vi "XW_Map_PreProc_wrapper_PN.vi"(4 "Domain padding factor":dbl=1.01, 6 "cap indicial sum to n":bool, 7 "XW_Calib_Map file path":path, 8 "surface order (n)":i32=3, 9 "Apply calibration corrections":bool=TRUE, 10 "Calib const":dbl[](array[numeric]) format="%.4f", 11 "Map method":T1=enum."Psi_eff, k = f(Umagn.)") -> ()   [LabVIEW 2010]
uses:
  XW calib map/Map method.ctl
  XW calib map/Qtree vis/Trimmed down TreeNode2D.ctl
  XW calib map/XW_Map_Global.vi
panel:
  out "All nodes processed and processed without error":bool
  # "For polysurface method only:"
  # "For trimesh method only:"
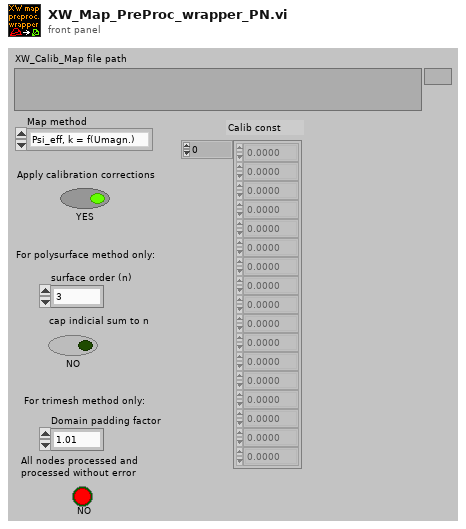
[diagram p1: front panel]
types:
  T1 = typedef "Map method.ctl" = enum16{"Triangle mesh", "Polynomial surface", "Const. Psi_eff (std.)", "Psi_eff = f(Umagn.)", "Psi_eff, k = f(Umagn.)"}
  T2 = cluster{"Calib const[0]":dbl, "Calib const[1]":dbl, "Calib const[2]":dbl, "Calib const[3]":dbl, "Calib const[4]":dbl, "Calib const[5]":dbl, "Calib const[6]":dbl, "Calib const[7]":dbl, "Calib const[8]":dbl, "Calib const[9]":dbl, "Calib const[10]":dbl, "Calib const[11]":dbl, "Calib const[12]":dbl, "Calib const[13]":dbl, "Calib const[14]":dbl, "Calib const[15]":dbl, "Calib const[16]":dbl, "Calib const[17]":dbl}
  T3 = typedef "Trimmed down TreeNode2D.ctl" = cluster{"Xmax":dbl, "Xmin":dbl, "Ymax":dbl, "Ymin":dbl, "Xc":dbl, "Yc":dbl, "ObjIndexList":i32[], "NodeQ1Index":i32, "NodeQ2Index":i32, "NodeQ3Index":i32, "NodeQ4Index":i32}
  T4 = typedef "Triangle2D.ctl" = cluster{"V10":dbl[], "V20":dbl[], "1/det":dbl, "V0":cluster{"PosVector":dbl[], "ValueVector":dbl[]}, "V1":cluster{"PosVector":dbl[], "ValueVector":dbl[]}, "V2":cluster{"PosVector":dbl[], "ValueVector":dbl[]}, "V21":dbl[]}
  T5 = typedef "TreeNode2D.ctl" = cluster{"Xmax":dbl, "Xmin":dbl, "Ymax":dbl, "Ymin":dbl, "Xc":dbl, "Yc":dbl, "Px":dbl, "Py":dbl, "q":dbl, "Level":i32, "ObjIndexList":i32[], "ParentIndex":i32, "NodeQ1Index":i32, "NodeQ2Index":i32, "NodeQ3Index":i32, "NodeQ4Index":i32, "EdgeVectorsQ1":dbl[][], "EdgeVectorsQ2":dbl[][], "EdgeVectorsQ3":dbl[][], "EdgeVectorsQ4":dbl[][], "PointOnEdgeVectorsQ1":dbl[][], "PointOnEdgeVectorsQ2":dbl[][], "PointOnEdgeVectorsQ3":dbl[][], "PointOnEdgeVectorsQ4":dbl[][]}
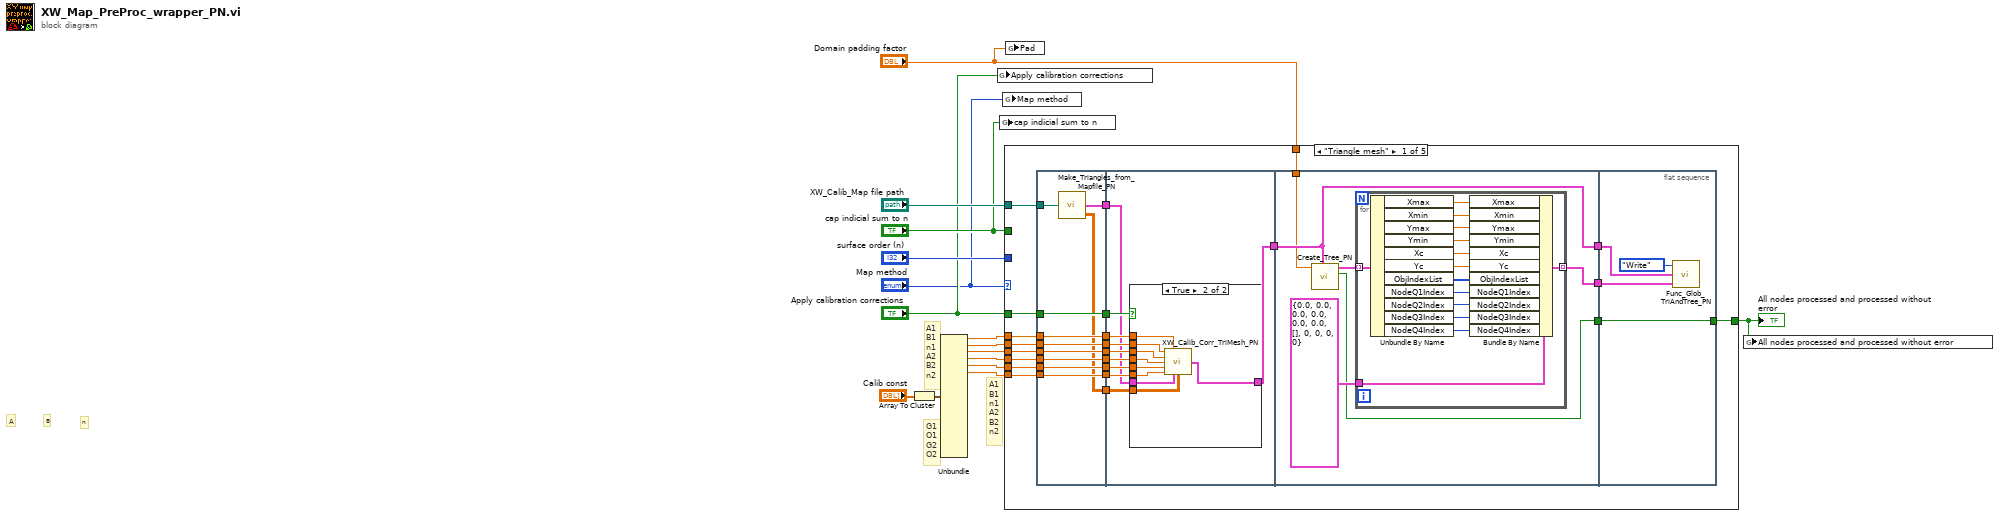
[diagram p0: block diagram]
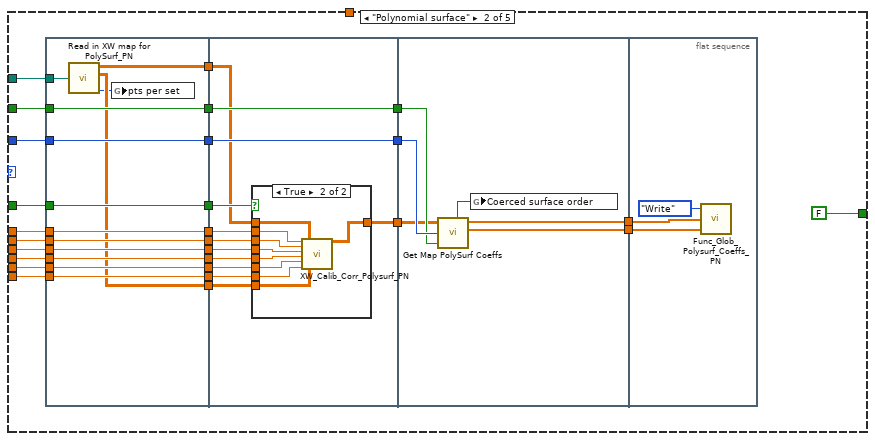
[diagram p3: hidden frame]
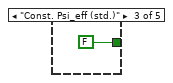
[diagram p5: hidden frame]
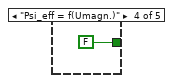
[diagram p6: hidden frame]
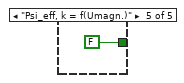
[diagram p7: hidden frame]
diagram:
  # "A1\nB1\nn1\nA2\nB2\nn2"
  # "G1\nO1\nG2\nO2"
  # "A1\nB1\nn1\nA2\nB2\nn2"
  # "n"
  # "B"
  # "A"
  n1 = Array To Cluster(array="Calib const") -> (cluster=w15:T2)
  n2 = Unbundle(w15) -> ("Calib const[0]"=w13:dbl, "Calib const[1]"=w12:dbl, "Calib const[2]"=w11:dbl, "Calib const[3]"=w10:dbl, "Calib const[4]"=w9:dbl, "Calib const[5]"=w8:dbl)  [unwired: 12 out]
  n3 = global write "XW_Map_Global.vi" "Apply calibration corrections"("Apply calibration corrections") -> ()
  n4 = global write "XW_Map_Global.vi" "cap indicial sum to n"("cap indicial sum to n") -> ()
  n5 = global write "XW_Map_Global.vi" "Map method"("Map method") -> ()
  n6 = case shown="\"Triangle mesh\"" "Map method" {
    tunnel: "Apply calibration corrections" -> [w38 w119 _ _ _]
    tunnel: w13 -> [w37 w118 _ _ _]
    tunnel: w12 -> [w36 w117 _ _ _]
    tunnel: w11 -> [w35 w116 _ _ _]
    tunnel: w10 -> [w34 w115 _ _ _]
    tunnel: w9 -> [w33 w114 _ _ _]
    tunnel: w8 -> [w32 w113 _ _ _]
    tunnel: "surface order (n)" -> [_ w112 _ _ _]
    tunnel: "cap indicial sum to n" -> [_ w111 _ _ _]
    tunnel: "XW_Calib_Map file path" -> [w31 w99 _ _ _]
    tunnel: [w23 FALSE FALSE ("All nodes processed and processed without error") FALSE ("All nodes processed and processed without error") FALSE ("All nodes processed and processed without error")] -> w1
    tunnel: "Domain padding factor" -> [w22 _ _ _ _]
    frame "Triangle mesh" {
      n7 = flat-sequence {
        tunnel: w31 -> [w41]
        tunnel: w32 -> [w42]
        tunnel: w33 -> [w43]
        tunnel: w34 -> [w44]
        tunnel: w35 -> [w45]
        tunnel: w36 -> [w46]
        tunnel: w37 -> [w47]
        tunnel: w38 -> [w48]
        tunnel: [w48] -> w30
        tunnel: [w47] -> w29
        tunnel: [w46] -> w28
        tunnel: [w45] -> w27
        tunnel: [w44] -> w26
        tunnel: [w43] -> w25
        tunnel: [w42] -> w24
        tunnel: [w40] -> w20
        tunnel: [w39] -> w16
        tunnel: w30 -> [w58]
        tunnel: w29 -> [w57]
        tunnel: w28 -> [w56]
        tunnel: w27 -> [w55]
        tunnel: w26 -> [w54]
        tunnel: w25 -> [w53]
        tunnel: w24 -> [w52]
        tunnel: w20 -> [w51]
        tunnel: [w50] -> w19
        tunnel: w16 -> [w49]
        tunnel: w22 -> [w69]
        tunnel: [w72] -> w21
        tunnel: w19 -> [w71]
        tunnel: [w71] -> w18
        tunnel: [w70] -> w17
        tunnel: [w92] -> w23
        tunnel: w21 -> [w92]
        tunnel: w18 -> [w91]
        tunnel: w17 -> [w90]
        frame #0 {
          n8 = call "Make_Triangles_from_Mapfile_PN.vi"("XW_Calib_Map file path (dialog if empty)"=w41) -> ("Triangles"=w40:T4[], "Zero angle dataset from map (used for calib. correction)"=w39:dbl[][])  [unwired: 1 out]
        }
        frame #1 {
          n9 = case shown="True" w58 {
            tunnel: w52 -> [_ w63]
            tunnel: w53 -> [_ w64]
            tunnel: w54 -> [_ w65]
            tunnel: w55 -> [_ w68]
            tunnel: w56 -> [_ w67]
            tunnel: w57 -> [_ w66]
            tunnel: w51 -> [w59 w62]
            tunnel: [w59 w61] -> w50
            tunnel: w49 -> [_ w60]
            frame False {
              # "if not correcting, then set\ncorrected tris equal to\noriginal tris for use"
            }
            frame True {
              n10 = call "XW_Calib_Corr_TriMesh_PN.vi"("B1 from Vel. Calib"=w67, "A1 from Vel. Calib"=w66, "n1 from Vel. Calib"=w68, "A2 from Vel. Calib"=w65, "B2 from Vel. Calib"=w64, "n2 from Vel. Calib"=w63, "Original triangles"=w62, "Zero angle dataset from map (used for calib. correction)"=w60) -> ("Corrected triangles"=w61:T4[])  [unwired: 7 out]
            }
          }
        }
        frame #2 {
          n11 = call "Create_Tree_PN.vi"("Triangles"=w71, "Pad"=w69) -> ("All nodes processed and processed without error"=w72:bool, "TreeNodes out"=w74:T5[])  [unwired: 3 in, 2 out]
          n12 = for {
            tunnel: w74 -> [w88] mode=indexing
            tunnel: [w86] -> w70 mode=indexing
            tunnel: T3 {"Xmax"=0.0, "Xmin"=0.0, "Ymax"=0.0, "Ymin"=0.0, "Xc"=0.0, "Yc"=0.0, "ObjIndexList"=[], "NodeQ1Index"=0, "NodeQ2Index"=0, "NodeQ3Index"=0, "NodeQ4Index"=0} ("Trimmed down TreeNode") -> [w87]
            n13 = Unbundle By Name(w88) -> ("Xmax"=w85:dbl, "Xmin"=w84:dbl, "Ymax"=w83:dbl, "Ymin"=w82:dbl, "Xc"=w81:dbl, "Yc"=w80:dbl, "ObjIndexList"=w79:i32[], "NodeQ1Index"=w78:i32, "NodeQ2Index"=w77:i32, "NodeQ3Index"=w76:i32, "NodeQ4Index"=w75:i32)
            n14 = Bundle By Name(cluster=w87, "Xmax"=w85, "Xmin"=w84, "Ymax"=w83, "Ymin"=w82, "Xc"=w81, "Yc"=w80, "ObjIndexList"=w79, "NodeQ1Index"=w78, "NodeQ2Index"=w77, "NodeQ3Index"=w76, "NodeQ4Index"=w75) -> (w86:T3)
          }
        }
        frame #3 {
          n15 = call "Func_Glob_TriAndTree_PN.vi"("Trimmed down TreeNode array IN"=w90, "Corrected triangles IN"=w91, "Action"=enum16{"Read", "Write"}."Write") -> ()  [unwired: 2 out]
        }
      }
    }
    frame "Polynomial surface" {
      n16 = flat-sequence {
        tunnel: w111 -> [w124]
        tunnel: w112 -> [w125]
        tunnel: w118 -> [w126]
        tunnel: w117 -> [w127]
        tunnel: w116 -> [w128]
        tunnel: w115 -> [w129]
        tunnel: w114 -> [w130]
        tunnel: w113 -> [w131]
        tunnel: w119 -> [w132]
        tunnel: [w132] -> w108
        tunnel: [w131] -> w107
        tunnel: [w130] -> w106
        tunnel: [w129] -> w105
        tunnel: [w128] -> w104
        tunnel: [w127] -> w103
        tunnel: [w126] -> w102
        tunnel: [w125] -> w101
        tunnel: [w124] -> w100
        tunnel: w99 -> [w123]
        tunnel: [w122] -> w97
        tunnel: [w121] -> w96
        tunnel: [w137] -> w110
        tunnel: [w136] -> w109
        tunnel: w108 -> [w144]
        tunnel: w107 -> [w138]
        tunnel: w106 -> [w139]
        tunnel: w105 -> [w140]
        tunnel: w104 -> [w141]
        tunnel: w103 -> [w142]
        tunnel: w102 -> [w143]
        tunnel: w101 -> [w137]
        tunnel: w100 -> [w136]
        tunnel: w97 -> [w135]
        tunnel: w96 -> [w134]
        tunnel: [w133] -> w95
        tunnel: w110 -> [w159]
        tunnel: w109 -> [w158]
        tunnel: w95 -> [w157]
        tunnel: [w156] -> w94
        tunnel: [w155] -> w93
        tunnel: w94 -> [w163]
        tunnel: w93 -> [w162]
        frame #0 {
          n17 = call "Read in XW map for PolySurf_PN.vi"("XW map file path (dialog if empty)"=w123) -> ("XW map values"=w122:dbl[][], "Zero angle dataset from map (used for calib. correction)"=w121:dbl[][], "pts per set"=w120:i32)  [unwired: 1 out]
          n18 = global write "XW_Map_Global.vi" "pts per set"(w120) -> ()
        }
        frame #1 {
          n19 = case shown="True" w144 {
            tunnel: w138 -> [_ w149]
            tunnel: w139 -> [_ w150]
            tunnel: w140 -> [_ w151]
            tunnel: w141 -> [_ w152]
            tunnel: w142 -> [_ w153]
            tunnel: w143 -> [_ w154]
            tunnel: w135 -> [w145 w148]
            tunnel: w134 -> [_ w147]
            tunnel: [w145 w146] -> w133
            frame False {
            }
            frame True {
              n20 = call "XW_Calib_Corr_Polysurf_PN.vi"("A1 from Vel. Calib"=w154, "B1 from Vel. Calib"=w153, "n1 from Vel. Calib"=w152, "A2 from Vel. Calib"=w151, "B2 from Vel. Calib"=w150, "n2 from Vel. Calib"=w149, "Original XW map values"=w148, "Zero angle dataset from map (used for calib. correction)"=w147) -> ("Corrected XW map values"=w146:dbl[][])  [unwired: 11 out]
            }
          }
        }
        frame #2 {
          n21 = call "Get Map PolySurf Coeffs.vi"("Corrected XW map values"=w157, "surface order (n)"=w159, "cap indicial sum to n"=w158) -> ("Ucal(m/s) coeffs"=w155:dbl[], "alpha(rad) coeffs"=w156:dbl[], "coerced surface order"=w160:i32)  [unwired: 2 out]
          n22 = global write "XW_Map_Global.vi" "Coerced surface order"(w160) -> ()
        }
        frame #3 {
          n23 = call "Func_Glob_Polysurf_Coeffs_PN.vi"("alpha(rad) coeffs IN"=w163, "Ucal coeffs IN"=w162, "Action"=enum16{"Read", "Write"}."Write") -> ()  [unwired: 2 out]
        }
      }
    }
    frame "Const. Psi_eff (std.)" {
    }
    frame "Psi_eff = f(Umagn.)" {
    }
    frame "Psi_eff, k = f(Umagn.)" {
    }
  }
  "All nodes processed and processed without error" <- w1
  n24 = global write "XW_Map_Global.vi" "Pad"("Domain padding factor") -> ()
  n25 = global write "XW_Map_Global.vi" "All nodes processed and processed without error"(w1) -> ()
